vi "DSF.Engine.Memory.Pointer.VS Channels.Data Ref to Pointer.vi"(8 "error in (no error)":errorcluster, 11 "Data Reference":T1 format="%.0x") -> (0 "error out":errorcluster, 3 "Channel Pointer":u64)   [LabVIEW 2016, in "DSF.Engine.lvlib" / "DSF.Engine.Memory.Pointer.VS Channels.lvclass"]
uses:
  DSF.Engine.Memory.Pointer.VS Channels.lvclass
  <vilib>/NI Veristand/Custom Device API/Data Reference.ctl
  <vilib>/NI Veristand/Custom Device API/Global Data Refs.vi
  <vilib>/NI Veristand/Custom Device API/Custom Device API.lvlib
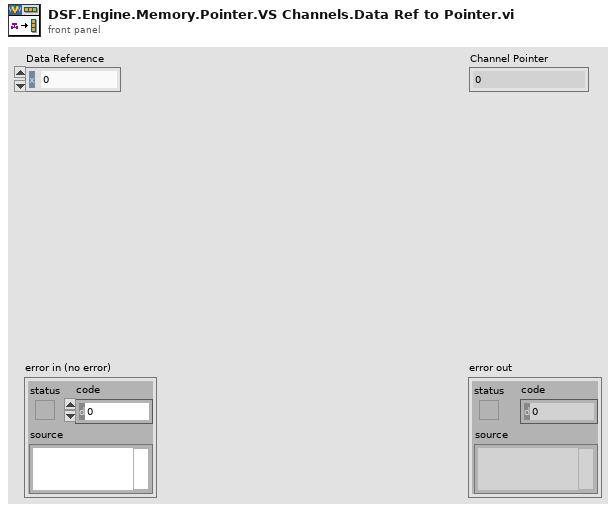
[diagram p1: front panel]
types:
  T1 = typedef "Custom Device API.lvlib/Data Reference.ctl" = i32
  T2 = typedef "Custom Device API.lvlib/Data Table Ref.ctl" = cluster{"Ptr.Beg":u64, "Ptr.End":u64}
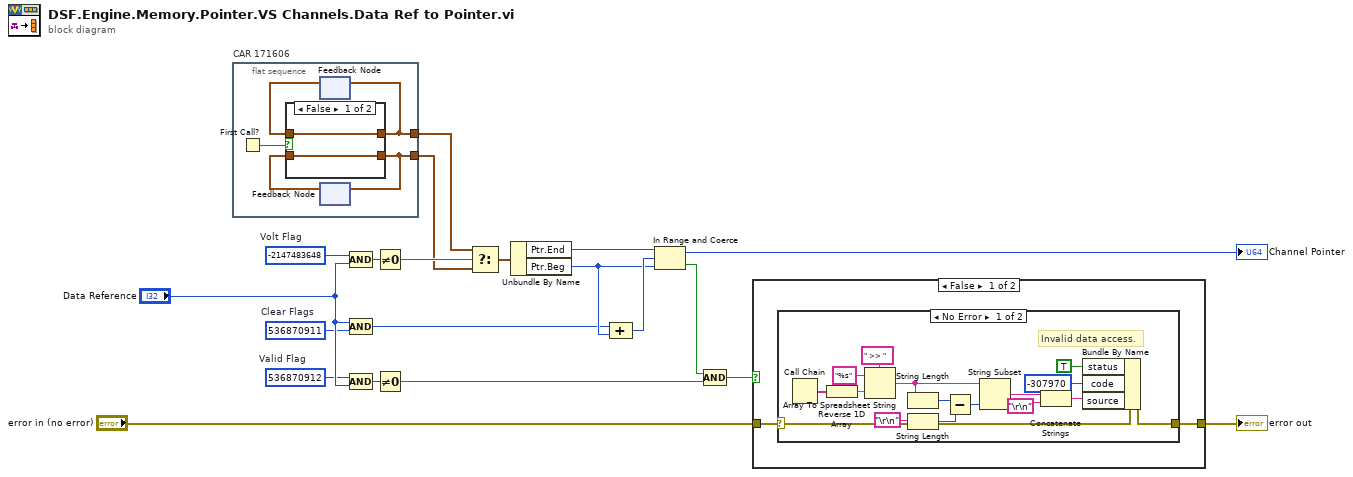
[diagram p0: block diagram]
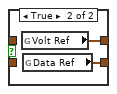
[diagram p2: hidden frame]
diagram:
  w7 = T1 536870912  # Valid Flag
  w8 = T1 536870911  # Clear Flags
  w9 = T1 -2147483648  # Volt Flag
  n1 = flat-sequence "CAR 171606" {
    tunnel: [w22] -> w6
    tunnel: [w21] -> w5
    frame #0 {
      n2 = First Call?() -> (First Call?: T/F=w25:bool)
      n3 = feedback #1() -> (w24:T2)  [unwired: 1 out]
      n4 = feedback #2() -> (w23:T2)  [unwired: 1 out]
      n5 = case shown="False" w25 {
        tunnel: [w27 w29] -> w22
        tunnel: w24 -> [w27 _]
        tunnel: [w26 w28] -> w21
        tunnel: w23 -> [w26 _]
        frame False {
        }
        frame True {
          n6 = global read "Global Data Refs.vi" "Volt Ref"() -> (w29:T2)
          n7 = global read "Global Data Refs.vi" "Data Ref"() -> (w28:T2)
        }
      }
      n8 = feedback-in #1(w22) -> ()
      n9 = feedback-in #2(w21) -> ()
    }
  }
  n10 = Compound Arithmetic op=AND(w9, "Data Reference") -> (w15:T1)
  n11 = Compound Arithmetic op=AND("Data Reference", w8) -> (w10:T1)
  n12 = Compound Arithmetic op=AND(w7, "Data Reference") -> (w12:T1)
  n13 = Not Equal To 0?(x=w15) -> (x != 0?=w14:bool)
  n14 = Not Equal To 0?(x=w12) -> (x != 0?=w11:bool)
  n15 = Select(t=w6, s=w14, f=w5) -> (s? t:f=w13:T2)
  n16 = Unbundle By Name(w13) -> ("Ptr.End"=w17:u64, "Ptr.Beg"=w16:u64)
  n17 = Compound Arithmetic op=ADD(w10, w16) -> (w19:u64)
  n18 = In Range and Coerce(upper limit=w17, x=w19, lower limit=w16) -> (coerced(x)=→"Channel Pointer":u64, In Range?=w18:bool)
  n19 = Compound Arithmetic op=AND(w18, w11) -> (w2:bool)
  n20 = case shown="False" w2 {
    tunnel: [w31 w49] -> w4
    tunnel: "error in (no error)" -> [w30 w49]
    frame False {
      n21 = case shown="No Error" w30 {
        selector: w30 -> [w44 w48]
        tunnel: [w47 w48] -> w31
        frame No Error {
          # "Invalid data access."
          n22 = Call Chain() -> (call chain=w33:string[])
          n23 = Reverse 1D Array(array=w33) -> (reversed array=w40:string[])
          n24 = Array To Spreadsheet String(delimiter (Tab)=" >> ", array=w40, 3:"%s" ("format string")) -> (spreadsheet string=w41:string)
          n25 = String Length(string=w41) -> (length=w39:i32)
          n26 = String Length(string="\r\n") -> (length=w43:i32)
          n27 = Subtract(x=w39, y=w43) -> (x-y=w38:i32)
          n28 = String Subset(string=w41, length (rest)=w38) -> (substring=w34:string)  [unwired: 1 out]
          n29 = Concatenate Strings(w34, "\r\n") -> (w32:string)
          n30 = Bundle By Name(cluster=w44, "status"=TRUE, "code"=-307970, "source"=w32) -> (w47:errorcluster)
        }
        frame Error {
          # "Leave existing error."
        }
      }
    }
    frame True {
    }
  }
  "error out" <- w4
